vi "WASD Keyboard Drive.vi"(7 "device ID":refnum<k1>) -> (0 "Y-Axis":dbl, 1 "X-Axis":dbl, 2 "key":T1(ring))   [LabVIEW 2013]
uses:
  <vilib>/Utility/inputDevices.llb/keyboardAcquire.vi
  <vilib>/Utility/inputDevices.llb/mouseAcquire.vi
panel:
  in  "Scrolling Down Constant":dbl
  out "Scrolling Down":dbl
  out "button 4":bool
  out "button 3":bool
  out "button 2":bool
  out "button 1":bool
  out "Horizontal Max":dbl
  in  "Scrolling Up Constant":dbl
  out "Vertical":dbl
  out "Horizontal":dbl
  out "Scrolling Up":dbl
  in  "mouse":bool
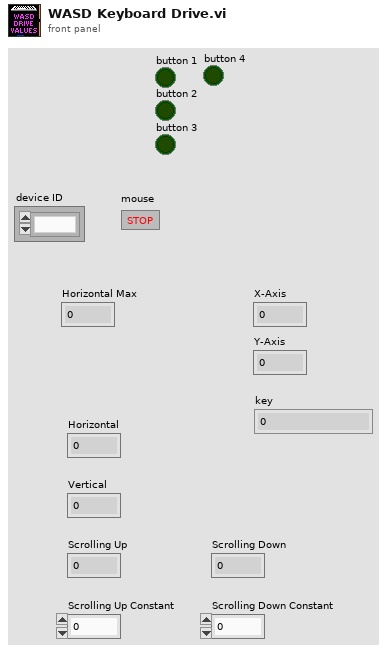
[diagram p1: front panel]
types:
  T1 = enum16{"0", "1", "2", "3", "4", "5", "6", "7", "8", "9", "A", "B", "C", "D", "E", "F", "G", "H", "I", "J", "K", "L", "M", "N", "O", "P", "Q", "R", "S", "T", "U", "V", "W", "X", "Y", "Z", "F1", "F2", "F3", "F4", "F5", "F6", "F7", "F8", "F9", "F10", "F11", "F12", "F13", "F14", "F15", "ADD", "BACK", "BACKSLASH", "CAPITAL", "COMMA", "DECIMAL", "DELETE", "DIVIDE", "DOWN", "END", "EQUALS", "ESCAPE", "GRAVE (`)", "HOME", "INSERT", "LBRACKET", "LCONTROL", "LEFT", "L ALT", "LSHIFT", "LWIN", "MINUS", "MULTIPLY", "NEXT", "NUMLOCK", "NUMPAD_0", "NUMPAD_1", "NUMPAD_2", "NUMPAD_3", "NUMPAD_4", "NUMPAD_5", "NUMPAD_6", "NUMPAD_7", "NUMPAD_8", "NUMPAD_9", "PAUSE", "PERIOD", "PRIOR (PG UP)", "RBRACKET", "RCONTROL", "RETURN", "RIGHT", "R ALT", "RSHIFT", "RWIN", "SCROLL", "SEMICOLON", "SLASH", "SPACE", "SUBTRACT", "TAB", "UP", "ENTER (num pad)", "' (quote)"}
  T2 = cluster{"Horizontal":i32, "Vertical":i32, "Scrolling":i32}
  T3 = cluster{"button 1":bool, "button 2":bool, "button 3":bool, "button 4":bool}
  T4 = enum16{"0", "1", "2", "3", "4", "5", "6", "7", "8", "9", "A", "B", "C", "D", "E", "F", "G", "H", "I", "J", "K", "L", "M", "N", "O", "P", "Q", "R", "S", "T", "U", "V", "W", "X", "Y", "Z", "F1", "F2", "F3", "F4", "F5", "F6", "F7", "F8", "F9", "F10", "F11", "F12", "F13", "F14", "F15", "ADD", "BACK", "BACKSLASH", "CAPITAL", "COMMA", "DECIMAL", "DELETE", "DIVIDE", "DOWN", "END", "EQUALS", "ESCAPE", "GRAVE (`)", "HOME", "INSERT", "LBRACKET", "LCONTROL", "LEFT", "L ALT", "LSHIFT", "LWIN", "MINUS", "MULTIPLY", "NEXT", "NUMLOCK", "NUMPAD_0", "NUMPAD_1", "NUMPAD_2", "NUMPAD_3", "NUMPAD_4", "NUMPAD_5", "NUMPAD_6", "NUMPAD_7", "NUMPAD_8", "NUMPAD_9", "PAUSE", "PERIOD", "PRIOR (PG UP)", "RBRACKET", "RCONTROL", "RETURN", "RIGHT", "R ALT", "RSHIFT", "RWIN", "SCROLL", "SEMICOLON", "SLASH", "SPACE", "SUBTRACT", "TAB", "UP", "ENTER (num pad)", "' (quote)"}[]
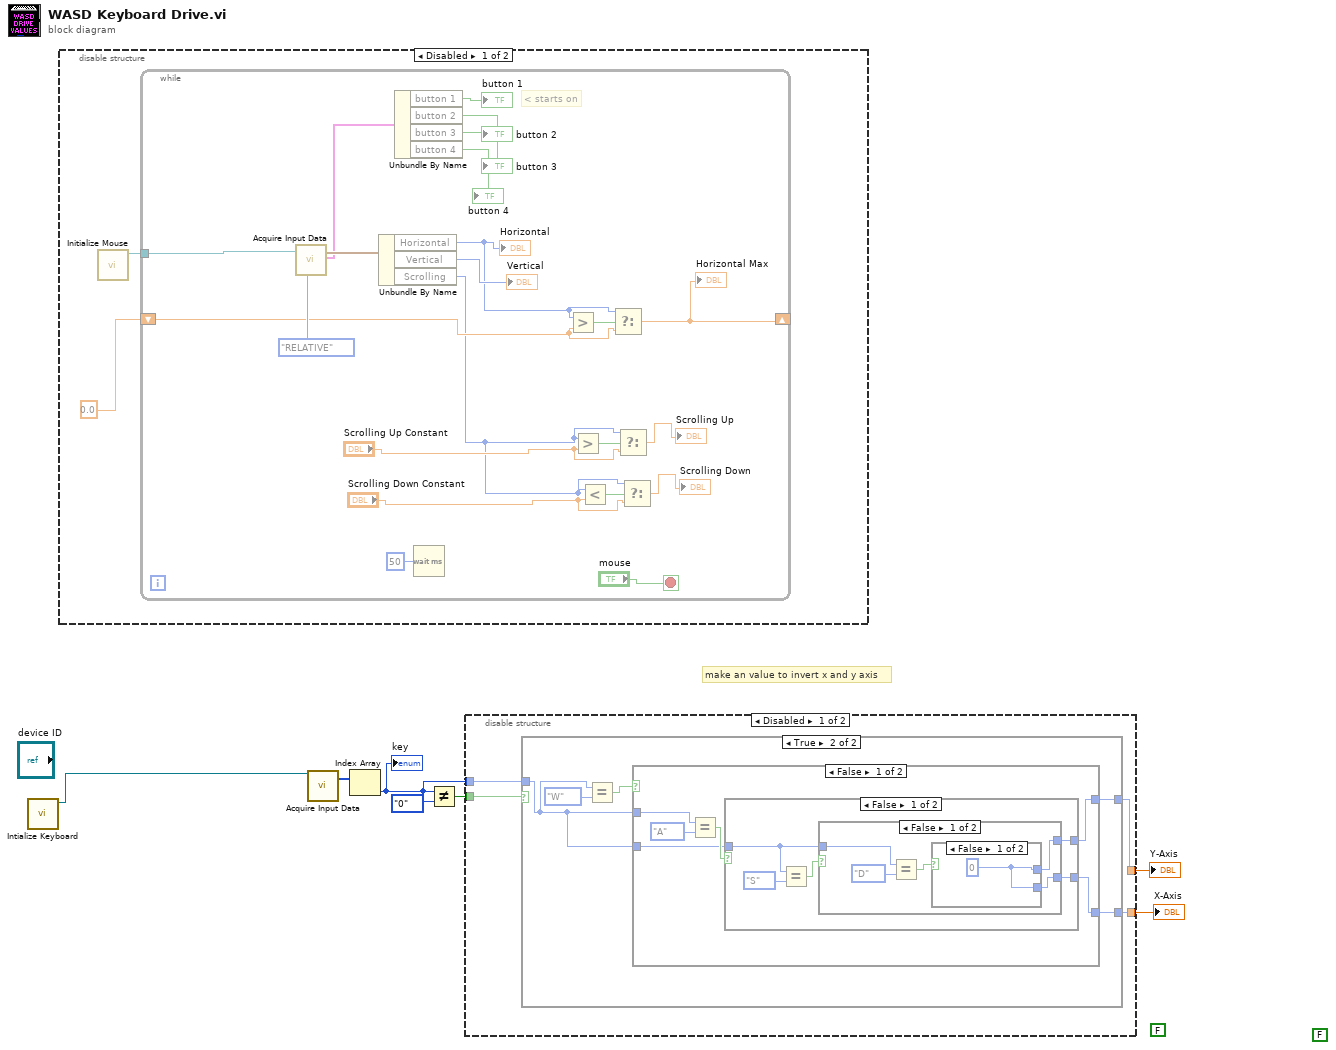
[diagram p0: block diagram]
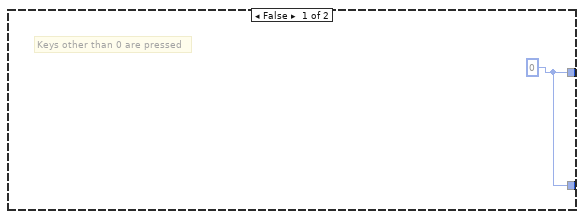
[diagram p2: hidden frame]
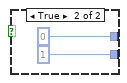
[diagram p3: hidden frame]
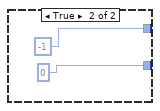
[diagram p4: hidden frame]
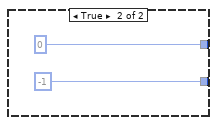
[diagram p5: hidden frame]
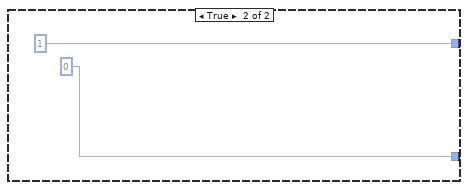
[diagram p6: hidden frame]
diagram:
  (unwired) FALSE
  (unwired) FALSE
  # "make an value to invert x and y axis"
  n1 = call <vilib>:"Intialize Keyboard.vi"() -> ("device ID"=w1:refnum<k1>)  [unwired: 10 in, 1 out]
  n2 = disable-structure shown="Disabled" {
    frame Disabled {
      n3 = call <vilib>:"Initialize Mouse.vi"() -> ("device ID"=w8:refnum<k1>)  [unwired: 10 in, 1 out]
      n4 = while {
        shift-right: [w19] -> _
        shift-left: 0.0 -> [w20]
        tunnel: w8 -> [w23]
        stop <- "mouse" stop-if-true
        # "< starts on"
        n5 = call-poly <vilib>:"Acquire Input Data.vi"("device ID"=w23, "key mode"=enum16{"RELATIVE", "ABSOLUTE"}."RELATIVE") -> ("axis info"=w24:T2, "button info"=w18:T3)  [unwired: 14 in, 2 out]
        n6 = Unbundle By Name(w24) -> ("Horizontal"=w21:i32, "Vertical"=→"Vertical":i32, "Scrolling"=w11:i32)
        "Horizontal" <- w21
        n7 = Unbundle By Name(w18) -> ("button 1"=→"button 1":bool, "button 2"=→"button 2":bool, "button 3"=→"button 3":bool, "button 4"=→"button 4":bool)
        n8 = Wait (ms)(milliseconds to wait=u32 50) -> ()  [unwired: 1 out]
        n9 = Greater?(x=w21, y=w20) -> (0:w22:bool)
        n10 = Greater?(x=w11, y="Scrolling Up Constant") -> (0:w28:bool)
        n11 = Less?(x=w11, y="Scrolling Down Constant") -> (x < y?=w12:bool)
        n12 = Select(t=w21, s=w22, f=w20) -> (s? t:f=w19:dbl)
        "Horizontal Max" <- w19
        n13 = Select(t=w11, s=w28, f="Scrolling Up Constant") -> (s? t:f=→"Scrolling Up":dbl)
        n14 = Select(t=w11, s=w12, f="Scrolling Down Constant") -> (s? t:f=→"Scrolling Down":dbl)
      }
    }
    frame Enabled {
    }
  }
  n15 = call-poly <vilib>:"Acquire Input Data.vi"("device ID"=w1) -> ("keys pressed"=w7:T4)  [unwired: 16 in, 2 out]
  n16 = Index Array(array=w7) -> (element=w4:T1)  [unwired: 1 in]
  "key" <- w4
  n17 = Not Equal?(x=w4, y=T1."0") -> (x != y?=w5:bool)
  n18 = disable-structure shown="Disabled" {
    disable-tunnel: w5 -> [w35 _]
    disable-tunnel: w4 -> [w34 _]
    disable-tunnel: [w33 _] -> w3
    disable-tunnel: [w32 _] -> w2
    frame Disabled {
      n19 = case shown="True" w35 {
        tunnel: w34 -> [_ w38]
        tunnel: [w36 w39] -> w33
        tunnel: [w36 w37] -> w32
        frame False {
          w36 = 0
          # "Keys other than 0 are pressed"
        }
        frame True {
          n20 = Equal?(x=w38, y=T1."W") -> (x = y?=w40:bool)
          n21 = case shown="False" w40 {
            tunnel: [w43 1] -> w39
            tunnel: w38 -> [w46 _]
            tunnel: w38 -> [w44 _]
            tunnel: [w42 0] -> w37
            frame False {
              n22 = Equal?(x=w46, y=T1."A") -> (x = y?=w45:bool)
              n23 = case shown="False" w45 {
                tunnel: w44 -> [w50 _]
                tunnel: [w49 0] -> w43
                tunnel: [w48 -1] -> w42
                frame False {
                  n24 = Equal?(x=w50, y=T1."S") -> (x = y?=w51:bool)
                  n25 = case shown="False" w51 {
                    tunnel: w50 -> [w56 _]
                    tunnel: [w54 -1] -> w49
                    tunnel: [w53 0] -> w48
                    frame False {
                      n26 = Equal?(x=w56, y=T1."D") -> (x = y?=w55:bool)
                      n27 = case shown="False" w55 {
                        tunnel: [w58 0] -> w54
                        tunnel: [w58 1] -> w53
                        frame False {
                          w58 = 0
                        }
                        frame True {
                        }
                      }
                    }
                    frame True {
                    }
                  }
                }
                frame True {
                }
              }
            }
            frame True {
            }
          }
        }
      }
    }
    frame Enabled {
    }
  }
  "Y-Axis" <- w3
  "X-Axis" <- w2
